vi "Read Measurement interval.vi"(8 "error in (no error)":errorcluster, 11 "EK-P4 in":refnum<class "EK-P4.lvclass">) -> (0 "error out":errorcluster, 2 "Measurement interval [ms]":u16=1, 3 "EK-P4 out":refnum<class "EK-P4.lvclass">)   [LabVIEW 2016, in "EK-P4.lvclass"]
doc: "read the measurment interval time in ms"
uses:
  EK-P4.lvclass
  EK-P4.lvclass/EK-P4.ctl
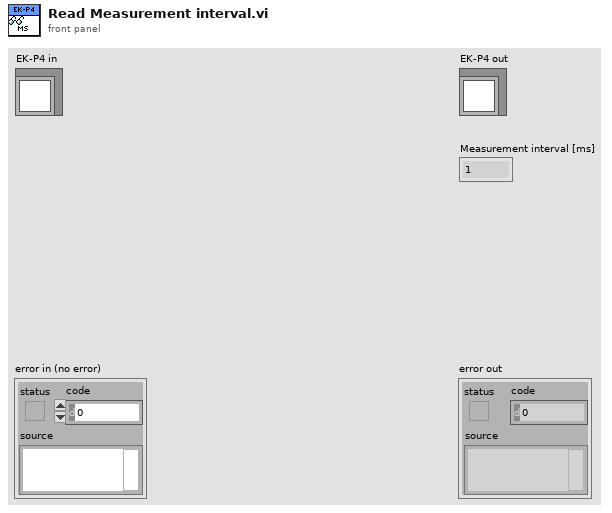
[diagram p1: front panel]
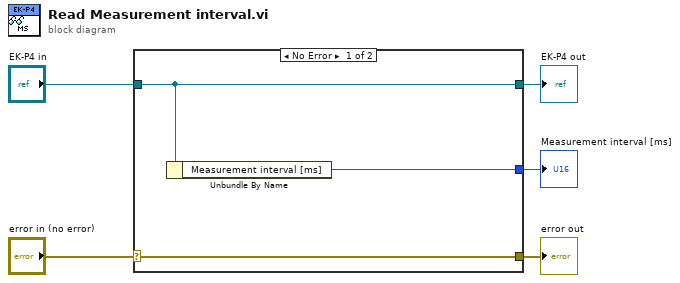
[diagram p0: block diagram]
diagram:
  n1 = case shown="No Error" "error in (no error)" {
    selector: "error in (no error)" -> [w8 w9]
    tunnel: [w8 w9] -> w4
    tunnel: [w7 w10] -> w2
    tunnel: "EK-P4 in" -> [w7 w10]
    tunnel: [w6 _] -> w1
    frame No Error {
      n2 = Unbundle By Name(w7) -> ("Measurement interval [ms]"=w6:u16)
    }
    frame Error {
    }
  }
  "error out" <- w4
  "EK-P4 out" <- w2
  "Measurement interval [ms]" <- w1
